vi "Page_Service_Config_WriteAll.vi"(6 "ctl references":T1, 8 "error in (no error)":errorcluster, 11 "AB_RESTfulWebService in":refnum<class "AB_RESTfulWebService.lvclass">) -> (0 "error out":errorcluster, 3 "AB_RESTfulWebService out":refnum<class "AB_RESTfulWebService.lvclass">)   [LabVIEW 2020, in "AB_RESTfulWebService.lvclass"]
uses:
  <vilib>/AppBuilder/AB_Classes/RESTful/AB_RESTfulWebService.lvclass
  <resource>/Framework/Providers/Builds/AppBuilder/AB_UI_Page_Service_Config_References.ctl
  <vilib>/AppBuilder/AB_Classes/RESTful/AB_RESTfulWebService.lvclass/AB_RESTfulWebService.ctl
  <vilib>/AppBuilder/AB_Classes/WebService/AB_WebService.lvclass
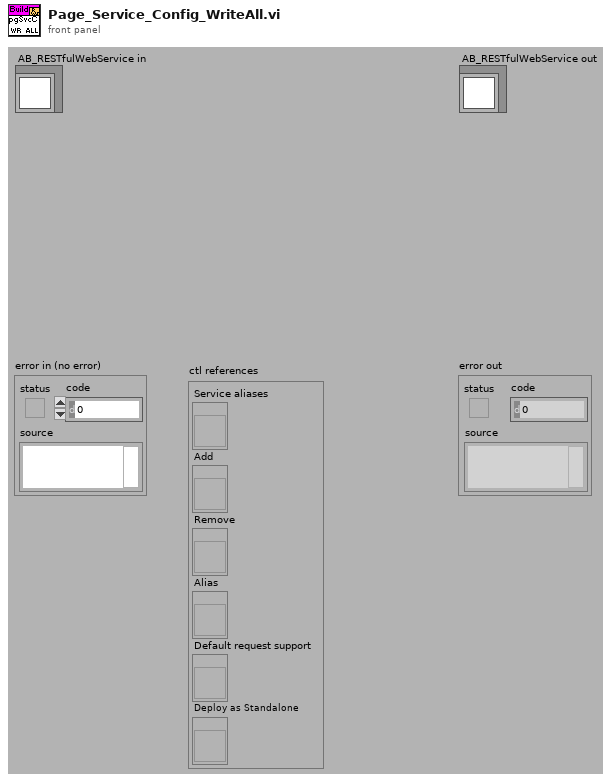
[diagram p1: front panel]
types:
  T1 = typedef "AB_UI_Page_Service_Config_References.ctl" = cluster{"Service aliases":refnum<vi>, "Add":refnum<vi>, "Remove":refnum<vi>, "Alias":refnum<vi>, "Default request support":refnum<vi>, "Deploy as Standalone":refnum<vi>}
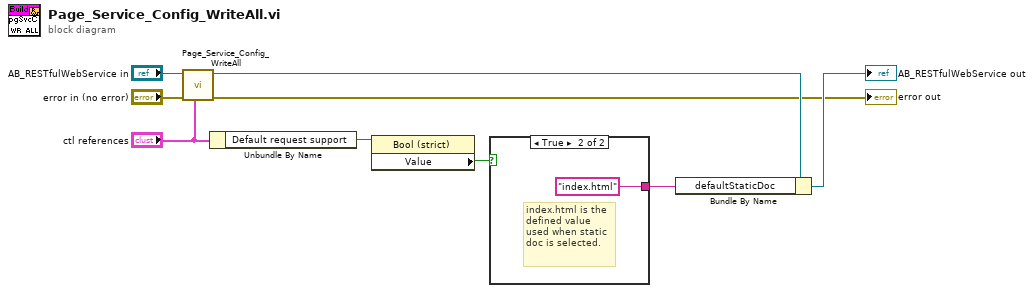
[diagram p0: block diagram]
diagram:
  n1 = call-parent "Page_Service_Config_WriteAll.vi"("ctl references"="ctl references", "error in (no error)"="error in (no error)", "AB_WebService in"="AB_RESTfulWebService in") -> ("error out"=→"error out":errorcluster, "AB_WebService out"=w7:refnum<class "AB_RESTfulWebService.lvclass">)  [unwired: 7 out]
  n2 = Unbundle By Name("ctl references") -> ("Default request support"=w4:refnum<vi>)
  n3 = property class="Bool (strict)"(reference=w4) -> ("Value"=w2:bool)  [unwired: 1 in, 2 out]
  n4 = case shown="True" w2 {
    tunnel: [_ "index.html"] -> w1
    frame False {
      # "Since option is not enabled, write out empty values."
    }
    frame True {
      # "index.html is the defined value used when static doc is selected."
    }
  }
  n5 = Bundle By Name(cluster=w7, "defaultStaticDoc"=w1) -> (→"AB_RESTfulWebService out":refnum<class "AB_RESTfulWebService.lvclass">)
